vi "Vacuum Test - Step 2.vi"(7 "Step":i32, 8 "error in":errorcluster, 9 "Test Results":T9, 10 "Oil In":T1, 11 "Test Configuration":T2) -> (0 "error out":errorcluster, 1 "Test Results Out":T9, 2 "Oil Out":T1, 3 "Test Configuration Out":T2)   [LabVIEW 2015]
uses:
  Controls/Test Results.ctl
  Controls/Step Result.ctl
  Controls/Startup Test.ctl
  Controls/Test Information.ctl
  Controls/Vacuum Test.ctl
  Controls/Test Timing.ctl
  Controls/Vaccum Thresholds.ctl
  Controls/Helium Test.ctl
  Controls/Helium Thresholds.ctl
  Controls/Startup Thresholds.ctl
  CAN Communication/Oil/Typedefs/Session Handle.ctl
  CAN Communication/Oil/Oil.lvclass
panel:
  out "NI-DAQ Pressure":dbl
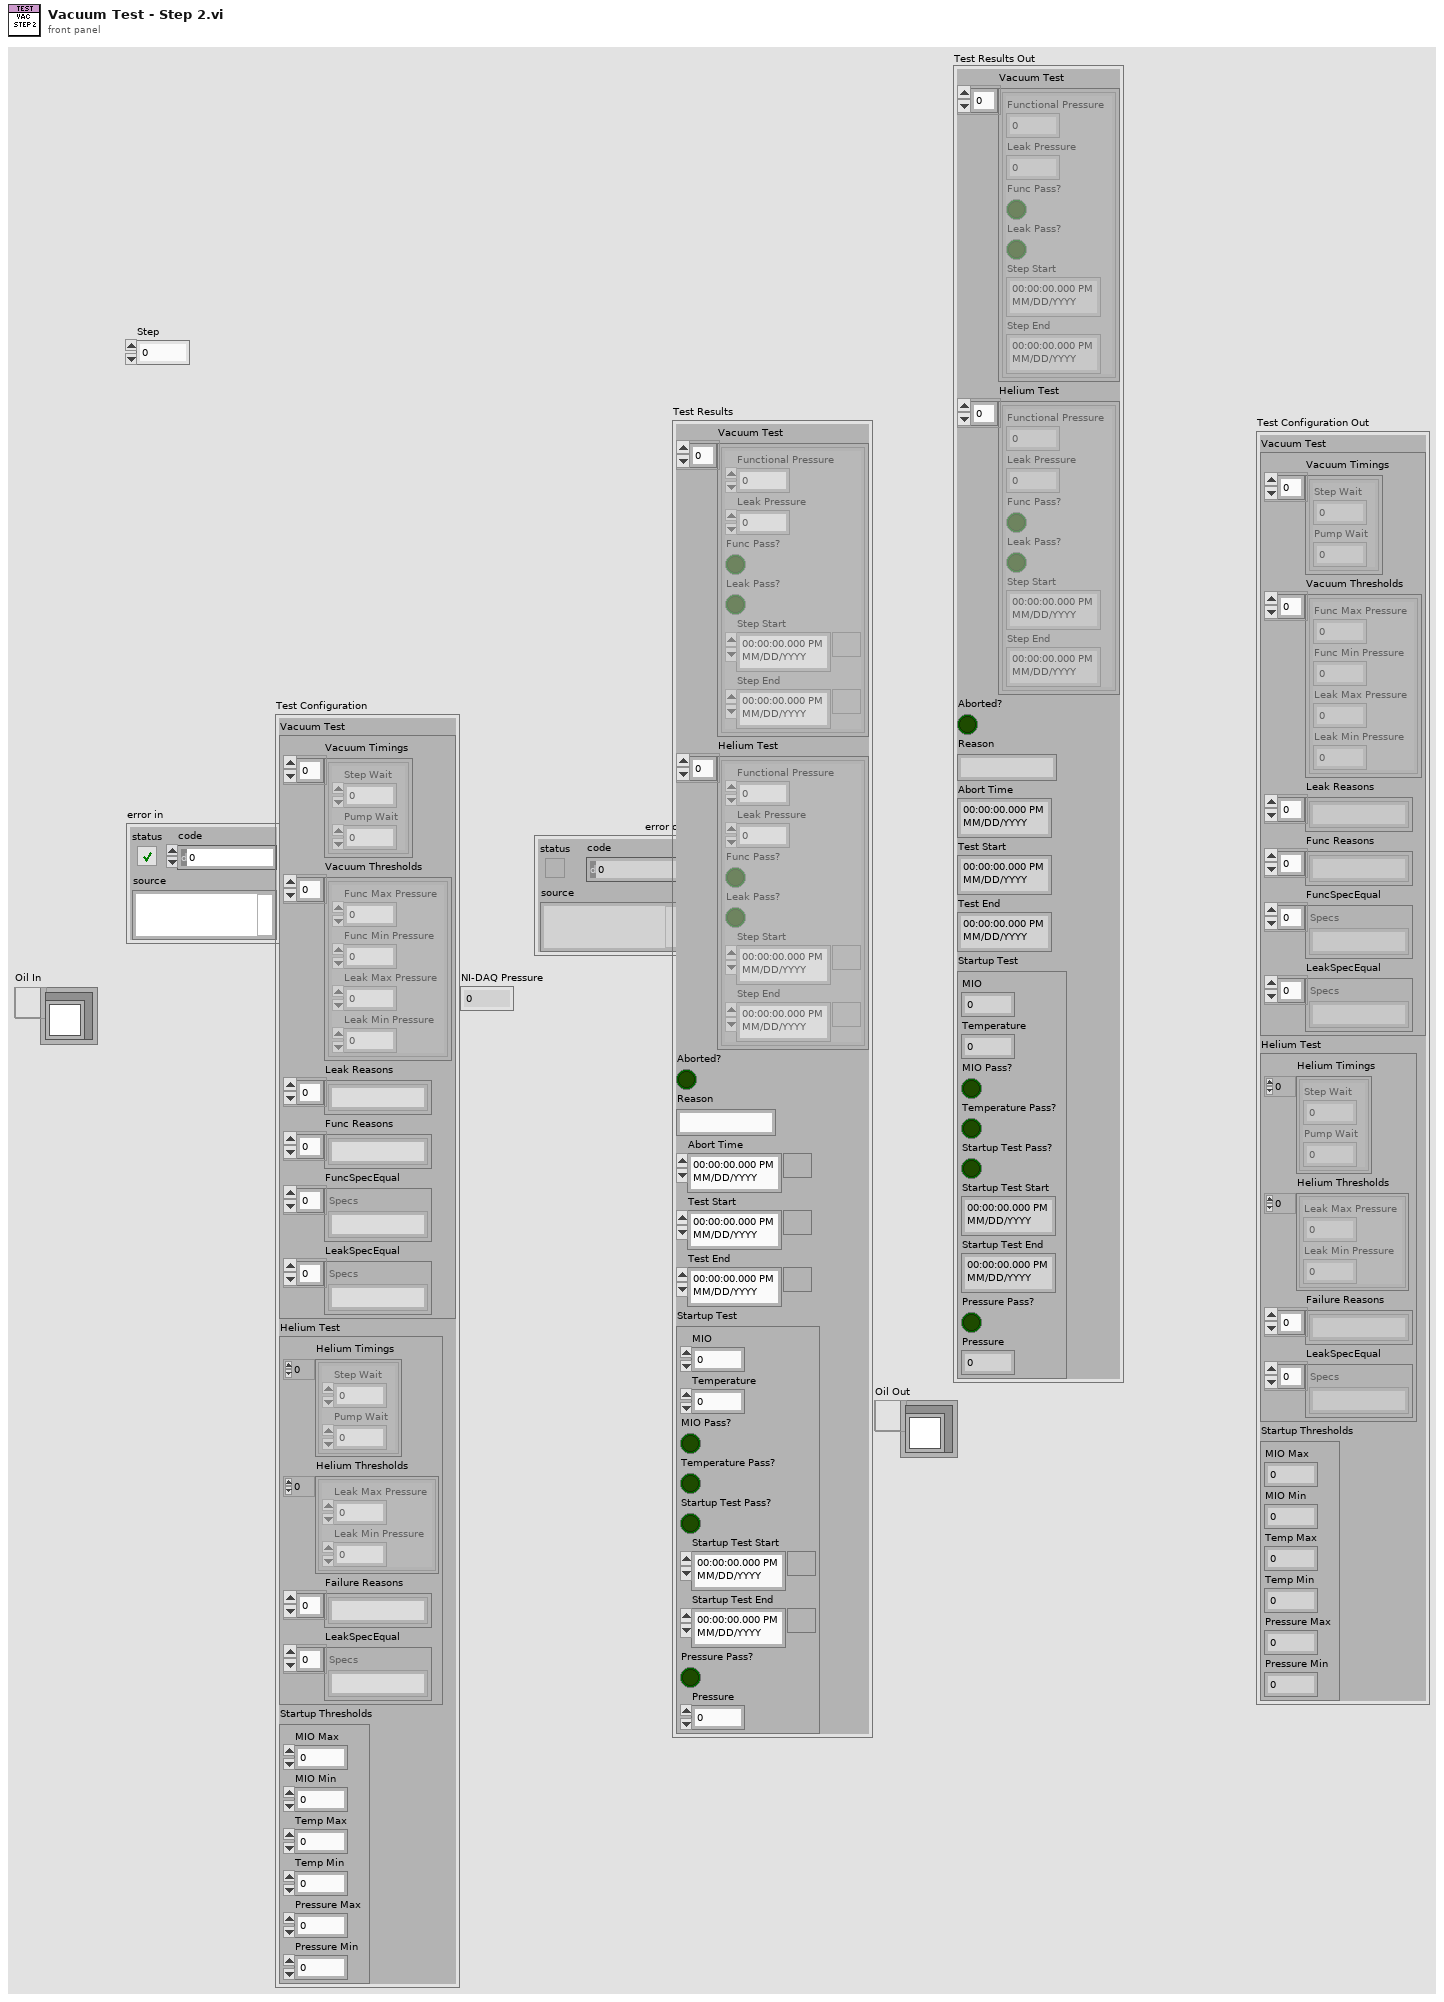
[diagram p1: front panel]
types:
  T1 = typedef "Oil.lvclass/Session Handle.ctl" = refnum<data-value>
  T2 = typedef "Test Information.ctl" = cluster{"Vacuum Test":T3, "Helium Test":T6, "Startup Thresholds":T8}
  T3 = typedef "Vacuum Test.ctl" = cluster{"Vacuum Timings":T4[], "Vacuum Thresholds":T5[], "Leak Reasons":string[], "Func Reasons":string[], "FuncSpecEqual":string[], "LeakSpecEqual":string[]}
  T4 = typedef "Test Timing.ctl" = cluster{"Step Wait":dbl, "Pump Wait":dbl}
  T5 = typedef "Vaccum Thresholds.ctl" = cluster{"Func Max Pressure":dbl, "Func Min Pressure":dbl, "Leak Max Pressure":dbl, "Leak Min Pressure":dbl}
  T6 = typedef "Helium Test.ctl" = cluster{"Helium Timings":T4[], "Helium Thresholds":T7[], "Failure Reasons":string[], "LeakSpecEqual":string[]}
  T7 = typedef "Helium Thresholds.ctl" = cluster{"Leak Max Pressure":dbl, "Leak Min Pressure":dbl}
  T8 = typedef "Startup Thresholds.ctl" = cluster{"MIO Max":dbl, "MIO Min":dbl, "Temp Max":dbl, "Temp Min":dbl, "Pressure Max":dbl, "Pressure Min":dbl}
  T9 = typedef "Test Results.ctl" = cluster{"Vacuum Test":T10[], "Helium Test":T10[], "Aborted?":bool, "Reason":string, "Abort Time":timestamp, "Test Start":timestamp, "Test End":timestamp, "Startup Test":T11}
  T10 = typedef "Step Result.ctl" = cluster{"Functional Pressure":dbl, "Leak Pressure":dbl, "Func Pass?":bool, "Leak Pass?":bool, "Step Start":timestamp, "Step End":timestamp}
  T11 = typedef "Startup Test.ctl" = cluster{"MIO":dbl, "Temperature":dbl, "MIO Pass?":bool, "Temperature Pass?":bool, "Startup Test Pass?":bool, "Startup Test Start":timestamp, "Startup Test End":timestamp, "Pressure Pass?":bool, "Pressure":dbl}
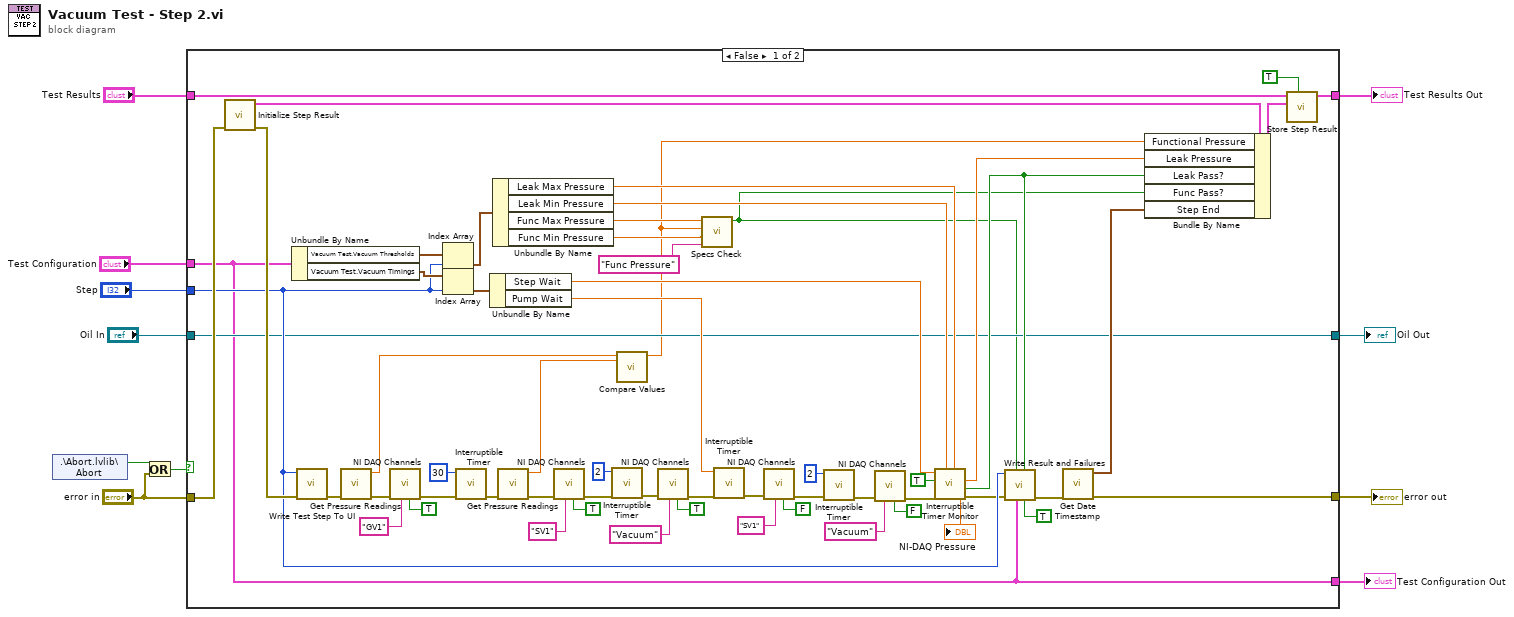
[diagram p0: block diagram]
diagram:
  n1 = shared-variable ".\\Abort.lvlib\\Abort"() -> (w10:bool)  [unwired: 1 in, 1 out]
  n2 = Or(x=w10, y="error in") -> (x .or. y?=w9:bool)
  n3 = case shown="False" w9 {
    tunnel: "error in" -> [w70 w73]
    tunnel: "Test Results" -> [w67 w74]
    tunnel: [w68 w74] -> w8
    tunnel: [w40 w73] -> w7
    tunnel: "Test Configuration" -> [w24 w72]
    tunnel: "Step" -> [w56 _]
    tunnel: [w24 w72] -> w3
    tunnel: [w41 w71] -> w1
    tunnel: "Oil In" -> [w41 w71]
    frame False {
      n4 = call "Initialize Step Result.vi"("error in (no error)"=w70) -> ("error out"=w69:errorcluster, "New Step Result"=w66:T10)  [unwired: 8 in, 1 out]
      n5 = Unbundle By Name(w24) -> ("Vacuum Test.Vacuum Thresholds"=w63:T5[], "Vacuum Test.Vacuum Timings"=w62:T4[])
      n6 = call "Write Test Step To UI.vi"("error in (no error)"=w69, "Step"=w56) -> ("error out"=w39:errorcluster)  [unwired: 9 in]
      n7 = call "Get Pressure Readings.vi"("error in (no error)"=w39) -> ("error out"=w37:errorcluster, "NI-DAQ Pressure"=w34:dbl)  [unwired: 7 in, 2 out]
      n8 = call "NI DAQ Channels.vi"("Control"=TRUE ("State"), "Channel"="GV1", "error in (no error)"=w37) -> ("error out"=w36:errorcluster)  [unwired: 7 in, 1 out]
      n9 = Index Array(array=w63, index=w56) -> (element=w57:T5)
      n10 = Index Array(array=w62, index=w56) -> (element=w61:T4)
      n11 = call "Interruptible Timer.vi"("error in (no error)"=w36, "Wait (s)"=30) -> ("error out"=w59:errorcluster)  [unwired: 7 in, 2 out]
      n12 = Unbundle By Name(w61) -> ("Step Wait"=w49:dbl, "Pump Wait"=w58:dbl)
      n13 = Unbundle By Name(w57) -> ("Leak Max Pressure"=w46:dbl, "Leak Min Pressure"=w47:dbl, "Func Max Pressure"=w16:dbl, "Func Min Pressure"=w15:dbl)
      n14 = call "Get Pressure Readings.vi"("error in (no error)"=w59) -> ("error out"=w32:errorcluster, "NI-DAQ Pressure"=w35:dbl)  [unwired: 7 in, 2 out]
      n15 = call "NI DAQ Channels.vi"("Control"=TRUE ("State"), "Channel"="SV1", "error in (no error)"=w32) -> ("error out"=w30:errorcluster)  [unwired: 7 in, 1 out]
      n16 = call "Interruptible Timer.vi"("error in (no error)"=w30, "Wait (s)"=2) -> ("error out"=w29:errorcluster)  [unwired: 7 in, 2 out]
      n17 = call "Compare Values.vi"("P2"=w35, "P1"=w34) -> ("Abs Diff"=w14:dbl)  [unwired: 9 in]
      n18 = call "NI DAQ Channels.vi"("Control"=TRUE ("State"), "Channel"="Vacuum", "error in (no error)"=w29) -> ("error out"=w52:errorcluster)  [unwired: 7 in, 1 out]
      n19 = call "Specs Check.vi"("parameter"="Func Pressure", "lower limit"=w15, "x"=w14, "upper limit"=w16) -> ("In Range?"=w12:bool)  [unwired: 6 in, 1 out]
      n20 = call "Interruptible Timer.vi"("error in (no error)"=w52, "Wait (s)"=w58) -> ("error out"=w28:errorcluster)  [unwired: 7 in, 2 out]
      n21 = call "NI DAQ Channels.vi"("Control"=FALSE ("State"), "Channel"="SV1", "error in (no error)"=w28) -> ("error out"=w26:errorcluster)  [unwired: 7 in, 1 out]
      n22 = call "Interruptible Timer.vi"("error in (no error)"=w26, "Wait (s)"=2) -> ("error out"=w27:errorcluster)  [unwired: 7 in, 2 out]
      n23 = call "NI DAQ Channels.vi"("Control"=FALSE ("State"), "Channel"="Vacuum", "error in (no error)"=w27) -> ("error out"=w50:errorcluster)  [unwired: 7 in, 1 out]
      n24 = call "Interruptible Timer Monitor.vi"("Max"=w46, "Min"=w47, "error in (no error)"=w50, "Update UI?"=TRUE, "Wait (s)"=w49) -> ("error out"=w43:errorcluster, "In Range?"=w44:bool, "Leak Rate"=w45:dbl, "NI-DAQ Pressure"=→"NI-DAQ Pressure":dbl)  [unwired: 2 in, 1 out]
      n25 = call "Write Result and Failures.vi"("Vacuum?"=TRUE, "Leak"=w44, "Test Configuration"=w24, "Func"=w12, "error in (no error)"=w43, "Step"=w56) -> ("error out"=w42:errorcluster)  [unwired: 5 in]
      n26 = call "Get Date Timestamp.vi"("error in (no error)"=w42) -> ("error out"=w40:errorcluster, "current time"=w64:timestamp)  [unwired: 9 in]
      n27 = Bundle By Name(cluster=w66, "Functional Pressure"=w14, "Leak Pressure"=w45, "Leak Pass?"=w44, "Func Pass?"=w12, "Step End"=w64) -> (w65:T10)
      n28 = call "Store Step Result.vi"("Vacuum?"=TRUE, "Step Result"=w65, "Test Results In"=w67) -> ("Test Results Out"=w68:T9)  [unwired: 8 in]
    }
    frame True {
    }
  }
  "error out" <- w7
  "Test Results Out" <- w8
  "Test Configuration Out" <- w3
  "Oil Out" <- w1
